vi "SMGR_intercom_03.vi"(8 "error in (no error)":errorcluster, 10 "InputData":T1={"DeviceID"=5, "DeviceDateTimeUTC"=timestamp(0 s since 1904-01-01), "log"=[], "SMGR2 FilePath"=path "D:/Work/SibNIIE/new_skil/skil/intercom/5-2012_07_18-00_32_53_4b.zip", "table FilePath"=path "D:/Work/SibNIIE/new_skil/skil/intercom/5-2012_07_18-00_32_53_4c.zip"}, 11 "URL:port":string="ssh.alwaysdata.com:12673") -> (0 "error out":errorcluster)   [LabVIEW 2010]
panel:
  out "answer":string
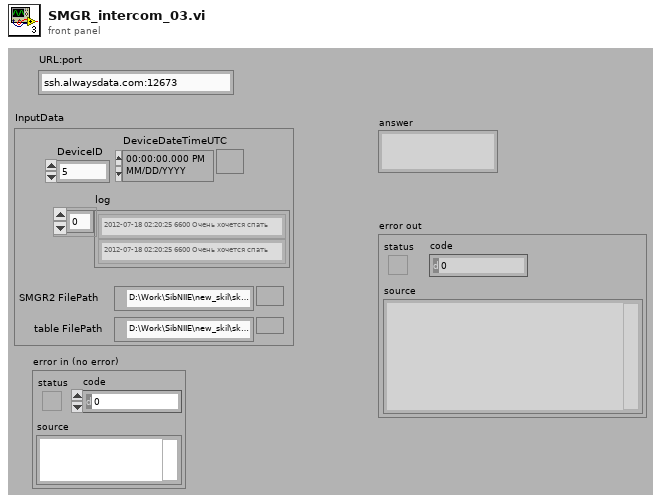
[diagram p1: front panel]
types:
  T1 = cluster{"DeviceID":i32, "DeviceDateTimeUTC":timestamp, "log":string[], "SMGR2 FilePath":path, "table FilePath":path}
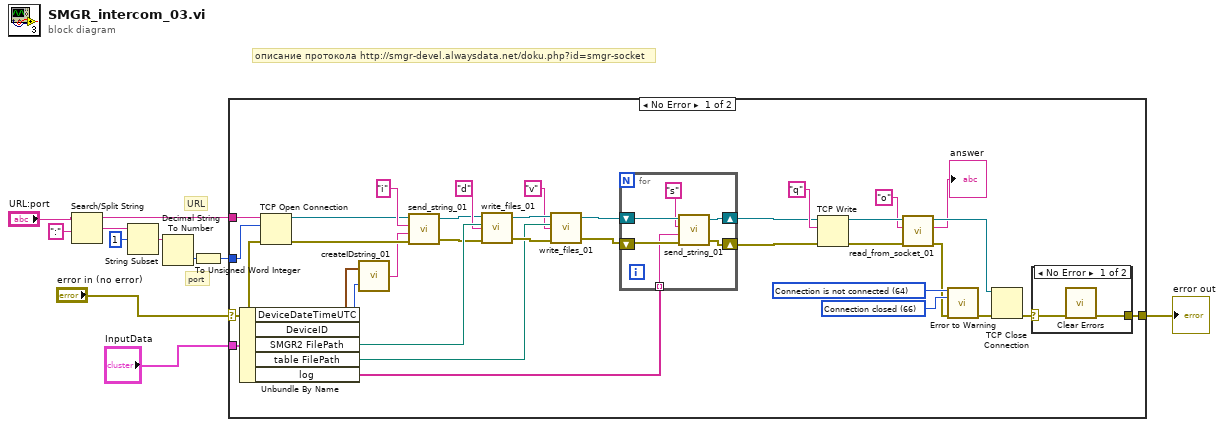
[diagram p0: block diagram]
diagram:
  # "описание протокола http://smgr-devel.alwaysdata.net/doku.php?id=smgr-socket"
  # "port"
  # "URL"
  n1 = Search/Split String(string="URL:port", search string/char (-)=":") -> (substring before match=w5:string, match + rest of string=w8:string)  [unwired: 1 in, 1 out]
  n2 = String Subset(string=w8, offset (0)=1) -> (substring=w9:string)  [unwired: 1 in]
  n3 = Decimal String To Number(string=w9) -> (number=w4:i32)  [unwired: 2 in, 1 out]
  n4 = To Unsigned Word Integer(number=w4) -> (unsigned 16bit integer=w2:u16)
  n5 = case shown="No Error" "error in (no error)" {
    selector: "error in (no error)" -> [w45 w56]
    tunnel: w5 -> [w46 _]
    tunnel: w2 -> [w44 _]
    tunnel: "InputData" -> [w32 _]
    tunnel: [w33 w56] -> w1
    frame No Error {
      w42 = 66 items=["No Error", "Argument Error", "Memory Full", "Out of Zone", "End of File", "File Already Open", "Generic File IO Error", "File Not Found", "File Permission Error", "Disk Full", "Duplicate Path", "Too Many Files Open", "Not Enabled", "Resource File Not Found", "Cannot Add Resource", "Resource Not Found", "Image Not Found", "Image Memory Error", "Pen Does Not Exist", "Config Bad Type", "Config Token Not Found", "Config Parse Error", "Config Memory Error", "Bad External Code Format", "Bad External Code Offset", "External Code Not Present", "Null Window", "Destroy Window Mixup", "Null Menu", "Print Aborted", "Bad Print Record", "Print Driver Error", "Windows Error During Print", "Memory Error During Print", "Print Dialog Error", "Generic Print Error", "Invalid Device Refnum", "Device Not Found", "Device Parameter Error", "Device Unit Error", "Can't Open Device", "Device Call Aborted", "Generic Error", "Cancelled By User", "Object ID Too Low", "Object ID Too High", "Object Not In Heap", "Unknown Heap", "Bad DefProc ID", "DefProc Not In Table", "Message Out Of Range", "Null Method", "Unknown Message", "Manager Call Not Supported", "Bad address", "Connection In progress", "Connection timed out", "Connection is already in progress", "Network attribute not supported", "Network error", "Address in use", "System out of memory", "Connection aborted", "Connection refused", "Connection is not connected", "Connection is already connected", "Connection closed", "Initialize error (interapplication manager)", "Bad occurrence", "Wait on unbound occurrence handler", "Occurrence queue overflow", "Bad path", "Semaphore not signaled", "Unrecognized type (interapplication manager)"] ("3rd Error to Convert")
      w43 = 64 items=["No Error", "Argument Error", "Memory Full", "Out of Zone", "End of File", "File Already Open", "Generic File IO Error", "File Not Found", "File Permission Error", "Disk Full", "Duplicate Path", "Too Many Files Open", "Not Enabled", "Resource File Not Found", "Cannot Add Resource", "Resource Not Found", "Image Not Found", "Image Memory Error", "Pen Does Not Exist", "Config Bad Type", "Config Token Not Found", "Config Parse Error", "Config Memory Error", "Bad External Code Format", "Bad External Code Offset", "External Code Not Present", "Null Window", "Destroy Window Mixup", "Null Menu", "Print Aborted", "Bad Print Record", "Print Driver Error", "Windows Error During Print", "Memory Error During Print", "Print Dialog Error", "Generic Print Error", "Invalid Device Refnum", "Device Not Found", "Device Parameter Error", "Device Unit Error", "Can't Open Device", "Device Call Aborted", "Generic Error", "Cancelled By User", "Object ID Too Low", "Object ID Too High", "Object Not In Heap", "Unknown Heap", "Bad DefProc ID", "DefProc Not In Table", "Message Out Of Range", "Null Method", "Unknown Message", "Manager Call Not Supported", "Bad address", "Connection In progress", "Connection timed out", "Connection is already in progress", "Network attribute not supported", "Network error", "Address in use", "System out of memory", "Connection aborted", "Connection refused", "Connection is not connected", "Connection is already connected", "Connection closed", "Initialize error (interapplication manager)", "Bad occurrence", "Wait on unbound occurrence handler", "Occurrence queue overflow", "Bad path", "Semaphore not signaled", "Unrecognized type (interapplication manager)"] ("1st Error to Convert")
      n6 = Unbundle By Name(w32) -> ("DeviceDateTimeUTC"=w18:timestamp, "DeviceID"=w19:i32, "SMGR2 FilePath"=w31:path, "table FilePath"=w29:path, "log"=w13:string[])
      n7 = TCP Open Connection(address=w46, remote port or service name=w44, error in (no error)=w45) -> (connection ID=w22:refnum<k5>, error out=w21:errorcluster)  [unwired: 2 in]
      n8 = call "createIDstring_01.vi"("DeviceID"=w19, "DateTime"=w18) -> ("result string"=w20:string)
      n9 = call "send_string_01.vi"("connection ID"=w22, "String flag (i s)"="i" ("FileFlag (d v)"), "Input string"=w20, "error out"=w21) -> ("connection ID 2"=w23:refnum<k5>, "error IO"=w24:errorcluster)  [unwired: 2 in]
      n10 = call "write_files_01.vi"("connection ID IN"=w23, "Path"=w31, "error in"=w24, "FileFlag (d v)"="d") -> ("connection ID Out"=w28:refnum<k5>, "error out"=w30:errorcluster)  [unwired: 2 in]
      n11 = call "write_files_01.vi"("connection ID IN"=w28, "Path"=w29, "error in"=w30, "FileFlag (d v)"="v") -> ("connection ID Out"=w16:refnum<k5>, "error out"=w17:errorcluster)  [unwired: 2 in]
      n12 = for {
        tunnel: w13 -> [w47] mode=indexing
        shift-right: [w49] -> w15
        shift-left: w16 -> [w51]
        shift-right: [w48] -> w14
        shift-left: w17 -> [w52]
        n13 = call "send_string_01.vi"("connection ID"=w51, "String flag (i s)"="s", "Input string"=w47, "error out"=w52) -> ("connection ID 2"=w49:refnum<k5>, "error IO"=w48:errorcluster)  [unwired: 2 in]
      }
      n14 = TCP Write(connection ID=w15, data in="q", error in (no error)=w14) -> (connection ID out=w38:refnum<k5>, error out=w39:errorcluster)  [unwired: 1 in, 1 out]
      n15 = call "read_from_socket_01.vi"("error out"=w39, "correct answer"="o", "In connection ID"=w38) -> ("warning out"=w35:errorcluster, "answer"=→"answer":string, "Out connection ID"=w36:refnum<k5>)  [unwired: 2 in]
      n16 = call <vilib>:"Error to Warning.vi"("1st Error to Convert"=w43, "2nd Error to Convert"=w42, "error in"=w35) -> ("warning out"=w41:errorcluster)  [unwired: 12 in]
      n17 = TCP Close Connection(connection ID=w36, error in (no error)=w41) -> (error out=w34:errorcluster)  [unwired: 1 in, 1 out]
      n18 = case shown="No Error" w34 {
        selector: w34 -> [w54 w55]
        tunnel: [w53 w55] -> w33
        frame No Error {
          n19 = call <vilib>:"Clear Errors.vi"("error in (no error)"=w54) -> ("error out"=w53:errorcluster)  [unwired: 6 in]
        }
        frame Error {
        }
      }
    }
    frame Error {
    }
  }
  "error out" <- w1
